vi "Sweep_Process.vi"(8 "错误输入（无错误）":errorcluster, 9 "MPM":refnum<k24>[](array[refnum]), 10 "TSL":refnum<k24>, 11 "SPU":refnum<k24>) -> (0 "error out":errorcluster, 1 "MPM out":refnum<k24>[](array[refnum]), 2 "TSL out":refnum<k24>, 3 "SPU out":refnum<k24>)   [LabVIEW 2017]
doc: "Sweep"
uses:
  D:/test/PDLSTS/LV_PDL LvVer17.0/LV_PDL_x86/DLL/InstrumentDLL.dll
  DLL/InstrumentDLL.dll
  Share/MPM_PowerMonitorType.vi
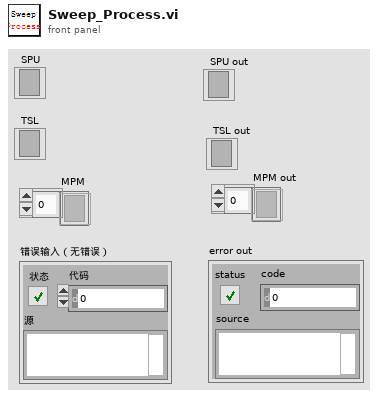
[diagram p1: front panel]
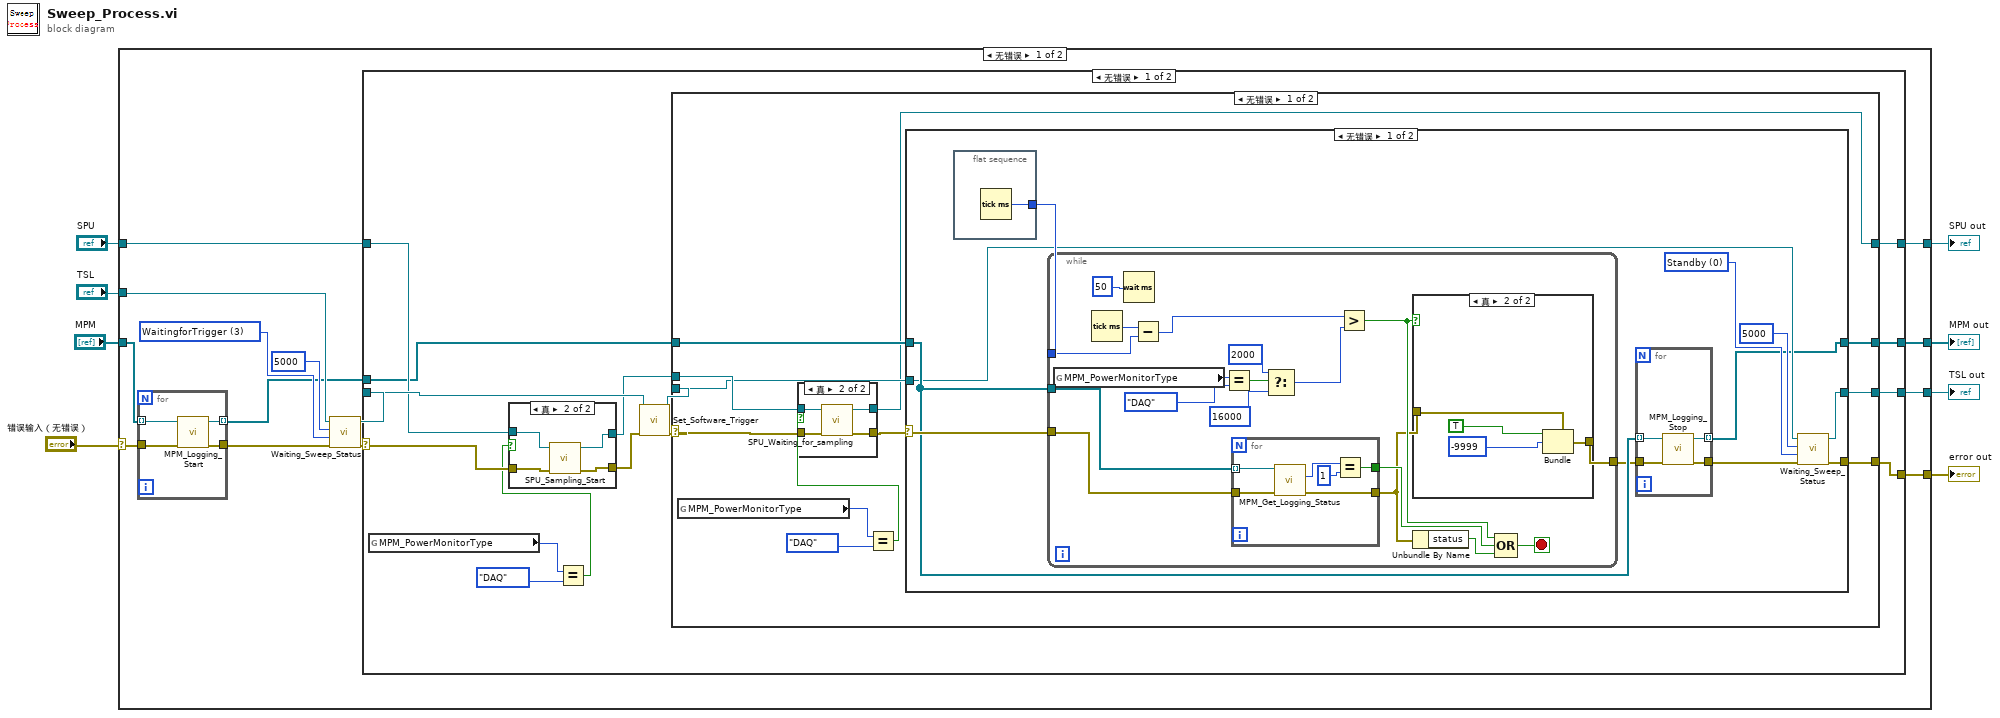
[diagram p0: block diagram]
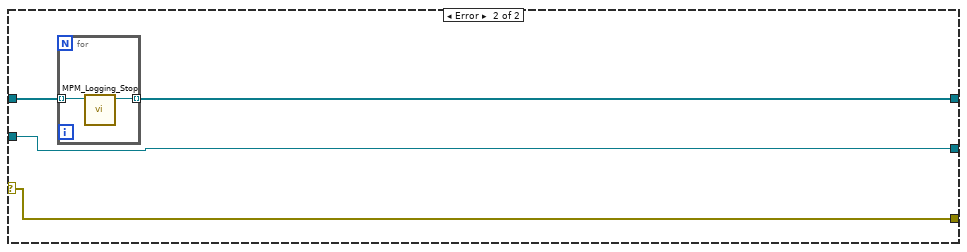
[diagram p5: hidden frame]
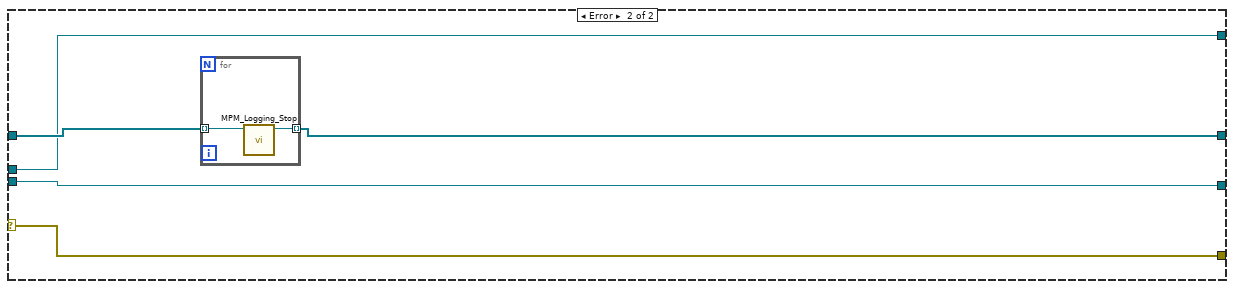
[diagram p6: hidden frame]
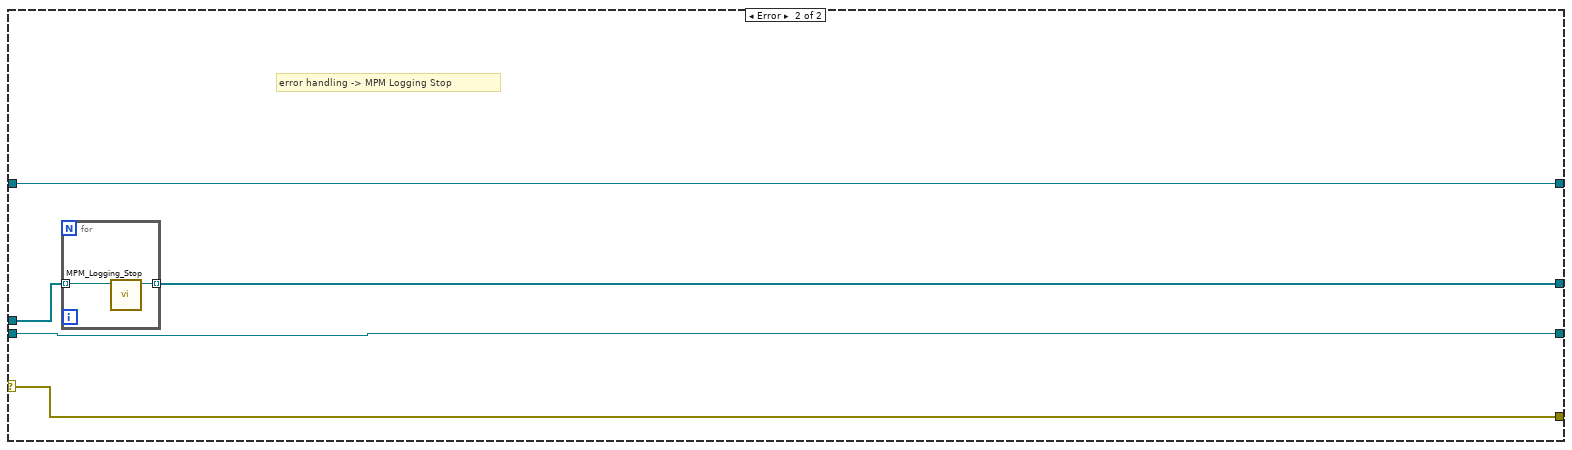
[diagram p7: hidden frame]
diagram:
  n1 = case shown="无错误" "错误输入（无错误）" {
    selector: "错误输入（无错误）" -> [w13 w134]
    tunnel: "SPU" -> [w22 w133]
    tunnel: "TSL" -> [w16 w132]
    tunnel: [w15 w134] -> w6
    tunnel: "MPM" -> [w14 w131]
    tunnel: [w12 w133] -> w3
    tunnel: [w11 w132] -> w2
    tunnel: [w9 w131] -> w1
    frame No Error {
      w19 = 3 items=["Standby", "Running", "Pausing", "WaitingforTrigger", "Returning"] ("status")
      n2 = for {
        tunnel: w14 -> [w130] mode=indexing
        tunnel: w13 -> [w129]
        tunnel: [w128] -> w17
        tunnel: [w127] -> w10 mode=indexing
        n3 = call "MPM_Logging_Start.vi"("error in (no error)"=w129, ".NET Reference in"=w130) -> ("error out"=w128:errorcluster, "Reference out"=w127:refnum<k24>)  [unwired: 8 in]
      }
      n4 = call "Waiting_Sweep_Status.vi"("error in (no error)"=w17, "status"=w19, "Wait time(msec)"=5000, ".NET Reference in"=w16) -> ("error out"=w20:errorcluster, "Reference out"=w21:refnum<k24>)  [unwired: 6 in]
      n5 = case shown="无错误" w20 {
        selector: w20 -> [w35 w123]
        tunnel: w21 -> [w36 w120]
        tunnel: w22 -> [w34 w122]
        tunnel: w10 -> [w33 w124]
        tunnel: [w29 w123] -> w15
        tunnel: [w28 w122] -> w12
        tunnel: [w27 w120] -> w11
        tunnel: [w26 w121] -> w9
        frame No Error {
          n6 = global read "MPM_PowerMonitorType.vi" "MPM_PowerMonitorType"() -> (w24:enum16{"DAQ", "MPM_220", "TSL_LOGG"})
          n7 = Equal?(x=w24, y=enum16{"DAQ", "MPM_220", "TSL_LOGG"}."DAQ") -> (x = y?=w23:bool)
          n8 = case shown="真" w23 {
            tunnel: [w38 w43] -> w37
            tunnel: w35 -> [w38 w42]
            tunnel: w34 -> [w39 w41]
            tunnel: [w39 w40] -> w31
            frame False {
            }
            frame True {
              n9 = call "SPU_Sampling_Start.vi"("错误输入（无错误）"=w42, "引用"=w41) -> ("error IO"=w43:errorcluster, "引用输出"=w40:refnum<k24>)  [unwired: 7 in]
            }
          }
          n10 = call "Set_Software_Trigger.vi"("error in (no error)"=w37, ".NET Reference in"=w36) -> ("error out"=w32:errorcluster, "Reference out"=w30:refnum<k24>)  [unwired: 8 in]
          n11 = case shown="无错误" w32 {
            selector: w32 -> [w55 w116]
            tunnel: w33 -> [w52 w117]
            tunnel: w31 -> [w54 w115]
            tunnel: w30 -> [w51 w113]
            tunnel: [w50 w116] -> w29
            tunnel: [w49 w115] -> w28
            tunnel: [w48 w113] -> w27
            tunnel: [w47 w114] -> w26
            frame No Error {
              n12 = global read "MPM_PowerMonitorType.vi" "MPM_PowerMonitorType"() -> (w46:enum16{"DAQ", "MPM_220", "TSL_LOGG"})
              n13 = Equal?(x=w46, y=enum16{"DAQ", "MPM_220", "TSL_LOGG"}."DAQ") -> (x = y?=w44:bool)
              n14 = case shown="真" w44 {
                tunnel: w55 -> [w56 w61]
                tunnel: w54 -> [w57 w60]
                tunnel: [w56 w59] -> w53
                tunnel: [w57 w58] -> w49
                frame False {
                }
                frame True {
                  n15 = call "SPU_Waiting_for_sampling.vi"("错误输入（无错误）"=w61, "引用"=w60) -> ("error IO"=w59:errorcluster, "引用输出"=w58:refnum<k24>)  [unwired: 7 in]
                }
              }
              n16 = case shown="无错误" w53 {
                selector: w53 -> [w72 w109]
                tunnel: w52 -> [w70 w110]
                tunnel: w51 -> [w66 w107]
                tunnel: [w65 w109] -> w50
                tunnel: [w63 w107] -> w48
                tunnel: [w62 w108] -> w47
                frame No Error {
                  w68 = 0 items=["Standby", "Running", "Pausing", "WaitingforTrigger", "Returning"] ("status")
                  n17 = flat-sequence {
                    tunnel: [w77] -> w71
                    frame #0 {
                      n18 = Tick Count (ms)() -> (millisecond timer value=w77:u32)
                    }
                  }
                  n19 = while {
                    tunnel: w70 -> [w95]
                    tunnel: w72 -> [w94]
                    tunnel: w71 -> [w91]
                    tunnel: [w84] -> w64
                    stop <- w88 stop-if-true
                    n20 = global read "MPM_PowerMonitorType.vi" "MPM_PowerMonitorType"() -> (w83:enum16{"DAQ", "MPM_220", "TSL_LOGG"})
                    n21 = Tick Count (ms)() -> (millisecond timer value=w92:u32)
                    n22 = Wait (ms)(milliseconds to wait=u32 50 ("等待时间（毫秒）")) -> ()  [unwired: 1 out]
                    n23 = Subtract(x=w92, y=w91) -> (x-y=w90:u32)
                    n24 = Equal?(x=w83, y=enum16{"DAQ", "MPM_220", "TSL_LOGG"}."DAQ") -> (x = y?=w81:bool)
                    n25 = for {
                      tunnel: w95 -> [w106] mode=indexing
                      tunnel: w94 -> [w105]
                      tunnel: [w102] -> w89
                      tunnel: [w101] -> w85
                      n26 = call "MPM_Get_Logging_Status.vi"("error in (no error)"=w105, ".NET Reference in"=w106) -> ("error out"=w101:errorcluster, "status out"=w104:i32)  [unwired: 6 in, 2 out]
                      n27 = Equal?(x=w104, y=1) -> (x = y?=w102:bool)
                    }
                    n28 = Select(t=2000, s=w81, f=16000) -> (s? t:f=w78:i32)
                    n29 = Greater?(x=w90, y=w78) -> (0:w86:bool)
                    n30 = case shown="真" w86 {
                      tunnel: w85 -> [w96 w100]
                      tunnel: [w96 w97] -> w84
                      frame False {
                      }
                      frame True {
                        n31 = Bundle(cluster=w100, "status"=TRUE, "code"=-9999) -> (w97:errorcluster)  [unwired: 1 in]
                      }
                    }
                    n32 = Unbundle By Name(w85) -> ("status"=w87:bool)
                    n33 = Compound Arithmetic op=OR ("复合运算")(w86, w89, w87) -> (w88:bool)
                  }
                  n34 = for {
                    tunnel: w70 -> [w76] mode=indexing
                    tunnel: [w75] -> w69
                    tunnel: w64 -> [w74]
                    tunnel: [w73] -> w62 mode=indexing
                    n35 = call "MPM_Logging_Stop.vi"("error in (no error)"=w74, ".NET Reference in"=w76) -> ("error out"=w75:errorcluster, "Reference out"=w73:refnum<k24>)  [unwired: 8 in]
                  }
                  n36 = call "Waiting_Sweep_Status.vi"("error in (no error)"=w69, "status"=w68, "Wait time(msec)"=5000, ".NET Reference in"=w66) -> ("error out"=w65:errorcluster, "Reference out"=w63:refnum<k24>)  [unwired: 6 in]
                }
                frame Error {
                  n37 = for {
                    tunnel: w110 -> [w112] mode=indexing
                    tunnel: [w111] -> w108 mode=indexing
                    n38 = call "MPM_Logging_Stop.vi"(".NET Reference in"=w112) -> ("Reference out"=w111:refnum<k24>)  [unwired: 9 in, 1 out]
                  }
                }
              }
            }
            frame Error {
              n39 = for {
                tunnel: w117 -> [w119] mode=indexing
                tunnel: [w118] -> w114 mode=indexing
                n40 = call "MPM_Logging_Stop.vi"(".NET Reference in"=w119) -> ("Reference out"=w118:refnum<k24>)  [unwired: 9 in, 1 out]
              }
            }
          }
        }
        frame Error {
          # "error handling -> MPM Logging Stop"
          n41 = for {
            tunnel: w124 -> [w126] mode=indexing
            tunnel: [w125] -> w121 mode=indexing
            n42 = call "MPM_Logging_Stop.vi"(".NET Reference in"=w126) -> ("Reference out"=w125:refnum<k24>)  [unwired: 9 in, 1 out]
          }
        }
      }
    }
    frame Error {
    }
  }
  "error out" <- w6
  "SPU out" <- w3
  "TSL out" <- w2
  "MPM out" <- w1
